vi "PRODUCT_COUNT_UPLOAD.vi"(8 "error in (no error)":errorcluster, 9 "Cluster":T1={"IP Address"=["", "", "", "", "", "", "", "", "", ""], "Machine name"=["", "", "", "", "", "", "", "", "", ""], "Station number"=["", "", "", "", "", "", "", "", "", ""], "Product List"=[], "Recipe_upload_history path"=path "", "reference"=refnum, "appended array"=[]}, 11 "CtlRef":refnum<vi>) -> (0 "error out":errorcluster, 1 "Quantity Day":i32[](array[numeric]), 5 "Quantity":string[](array[string]))   [LabVIEW 2017]
uses:
  Controls/cluster.ctl
  <vilib>/addons/database/Connection.llb/Conn ObjectReference.ctl
  <vilib>/addons/database/NI_Database_API.lvlib
panel:
  in  "Quantity PER DAYS":i32
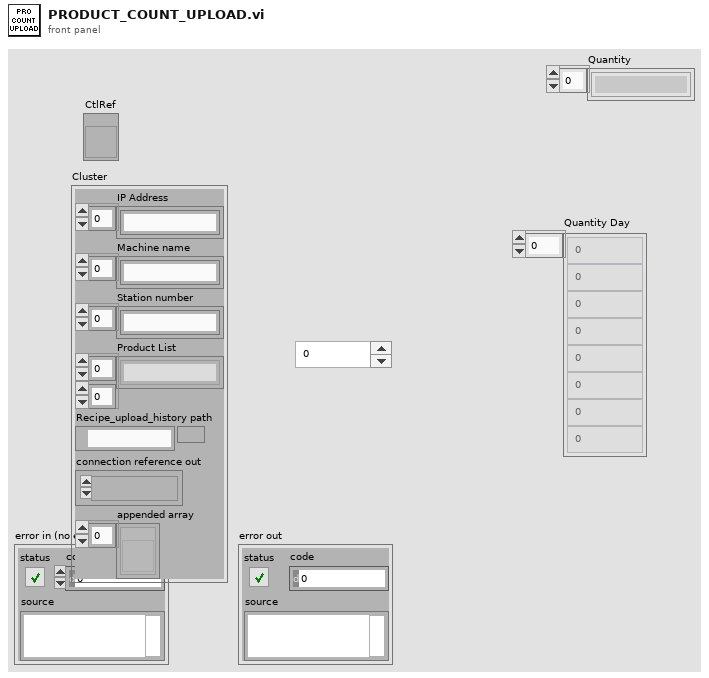
[diagram p1: front panel]
types:
  T1 = typedef "cluster.ctl" = cluster{"IP Address":string[], "Machine name":string[], "Station number":string[], "Product List":string[][], "Recipe_upload_history path":path, "reference":T2, "appended array":refnum<vi>[]}
  T2 = typedef "NI_Database_API.lvlib/Conn ObjectReference.ctl" = refnum<k1>
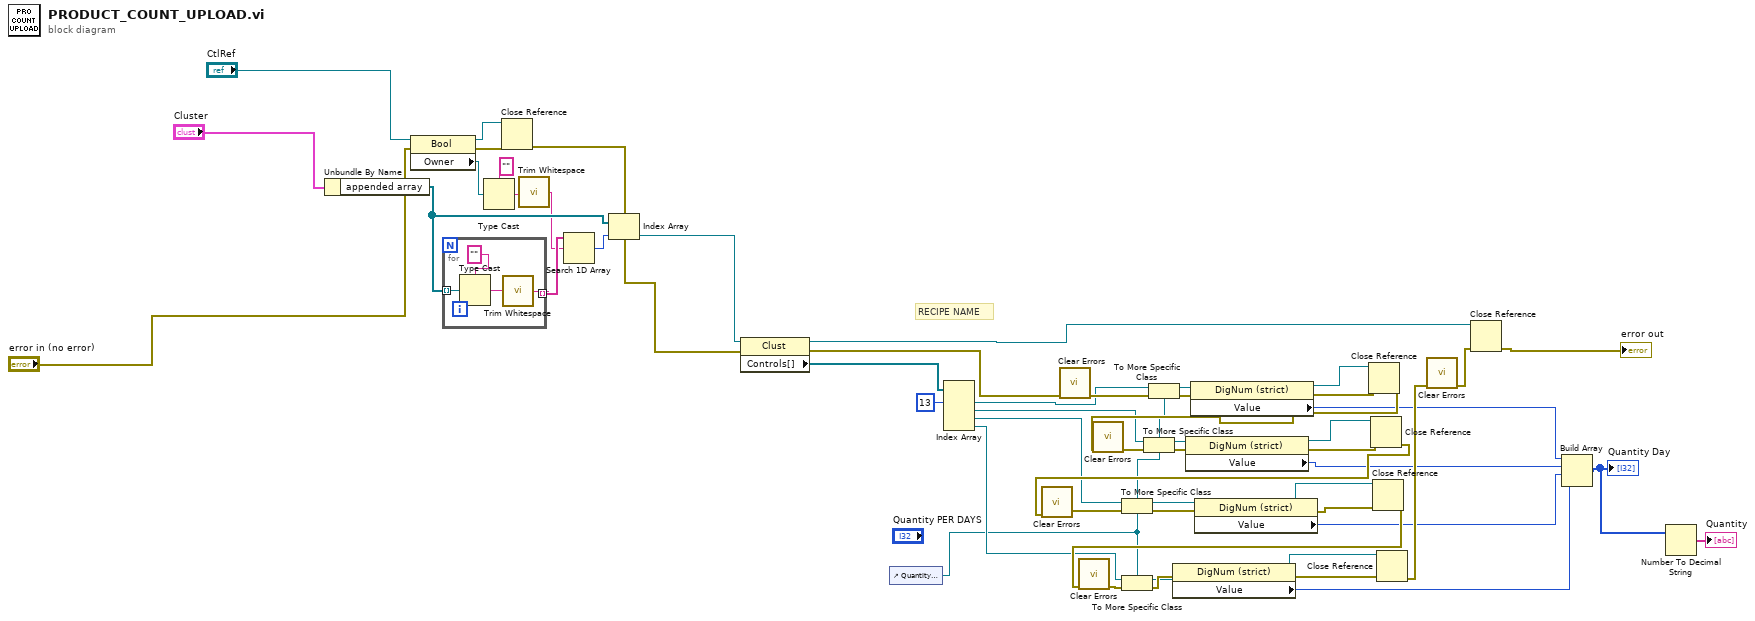
[diagram p0: block diagram]
diagram:
  # "RECIPE NAME"
  n1 = Unbundle By Name("Cluster") -> ("appended array"=w54:refnum<vi>[])
  n2 = property class="Bool"(reference="CtlRef", error in="error in (no error)") -> (reference out=w46:refnum<vi>, error out=w47:errorcluster, "Owner"=w50:refnum<vi>)
  n3 = for {
    tunnel: w54 -> [w59] mode=indexing
    tunnel: [w56] -> w52 mode=indexing
    n4 = Type Cast(type="" ("String"), x=w59) -> (*(type *) &x=w57:string)
    n5 = call <vilib>:"Trim Whitespace.vi"("string"=w57) -> ("trimmed string"=w56:string)  [unwired: 1 in]
  }
  n6 = Type Cast(type="", x=w50) -> (*(type *) &x=w49:string)
  n7 = Close Reference(reference=w46, error in (no error)=w47) -> (error out=w8:errorcluster)
  n8 = call <vilib>:"Trim Whitespace.vi"("string"=w49) -> ("trimmed string"=w51:string)  [unwired: 1 in]
  n9 = Search 1D Array(1D array=w52, element=w51) -> (index of element=w53:i32)  [unwired: 1 in]
  n10 = Index Array(array=w54, index=w53) -> (element=w10:refnum<vi>)
  n11 = property class="Clust"(reference=w10, error in=w8) -> (reference out=w42:refnum<vi>, error out=w43:errorcluster, "Controls[]"=w40:refnum<vi>[])
  n12 = control-ref of="Quantity PER DAYS"() -> (w3:refnum<vi>)
  n13 = Index Array(array=w40, index #1=13 ("index")) -> (element #1=w16:refnum<vi>, element #2=w20:refnum<vi>, element #3=w25:refnum<vi>, element #4=w11:refnum<vi>)  [unwired: 3 in]
  n14 = call <vilib>:"Clear Errors.vi"("error in (no error)"=w43) -> ("error out"=w19:errorcluster)  [unwired: 5 in, 1 out]
  n15 = To More Specific Class(target class=w3, reference=w16, error in=w19) -> (specific class reference=w17:refnum<vi>, error out=w18:errorcluster)
  n16 = property class="DigNum (strict)"(reference=w17, error in=w18) -> (reference out=w33:refnum<vi>, error out=w41:errorcluster, "Value"=w7:i32)
  n17 = Close Reference(reference=w33, error in (no error)=w41) -> (error out=w36:errorcluster)
  n18 = call <vilib>:"Clear Errors.vi"("error in (no error)"=w36) -> ("error out"=w23:errorcluster)  [unwired: 5 in, 1 out]
  n19 = To More Specific Class(target class=w3, reference=w20, error in=w23) -> (specific class reference=w21:refnum<vi>, error out=w22:errorcluster)
  n20 = property class="DigNum (strict)"(reference=w21, error in=w22) -> (reference out=w32:refnum<vi>, error out=w38:errorcluster, "Value"=w6:i32)
  n21 = Close Reference(reference=w32, error in (no error)=w38) -> (error out=w35:errorcluster)
  n22 = call <vilib>:"Clear Errors.vi"("error in (no error)"=w35) -> ("error out"=w26:errorcluster)  [unwired: 5 in, 1 out]
  n23 = To More Specific Class(target class=w3, reference=w25, error in=w26) -> (specific class reference=w24:refnum<vi>, error out=w27:errorcluster)
  n24 = property class="DigNum (strict)"(reference=w24, error in=w27) -> (reference out=w31:refnum<vi>, error out=w37:errorcluster, "Value"=w5:i32)
  n25 = Close Reference(reference=w31, error in (no error)=w37) -> (error out=w34:errorcluster)
  n26 = call <vilib>:"Clear Errors.vi"("error in (no error)"=w34) -> ("error out"=w29:errorcluster)  [unwired: 5 in, 1 out]
  n27 = To More Specific Class(target class=w3, reference=w11, error in=w29) -> (specific class reference=w15:refnum<vi>, error out=w28:errorcluster)
  n28 = property on="Property Node" class="DigNum (strict)"(reference=w15, error in=w28) -> (reference out=w30:refnum<vi>, error out=w12:errorcluster, "Value"=w4:i32)
  n29 = Close Reference(reference=w30, error in (no error)=w12) -> (error out=w14:errorcluster)
  n30 = call <vilib>:"Clear Errors.vi"("error in (no error)"=w14) -> ("error out"=w13:errorcluster)  [unwired: 5 in, 1 out]
  n31 = Close Reference(reference=w42, error in (no error)=w13) -> (error out=→"error out":errorcluster)
  n32 = Build Array(w7, w6, w5, w4) -> (w2:i32[])
  "Quantity Day" <- w2
  n33 = Number To Decimal String(number=w2) -> (decimal integer string=→"Quantity":string[])  [unwired: 1 in]
